vi "Reset.vi"(8 "error in (no error)":errorcluster, 10 "Set Defaults? (F)":bool, 11 "VISA resource name":refnum<visa-resource-name>) -> (0 "error out":errorcluster, 3 "VISA resource name out":refnum<visa-resource-name>)   [LabVIEW 2011, in "MGC647C.lvlib"]
doc: "Resets the instrument and then sends a set of default setup commands to the instrument."
uses:
  <instrlib>/MGC647C/MGC647C.lvlib
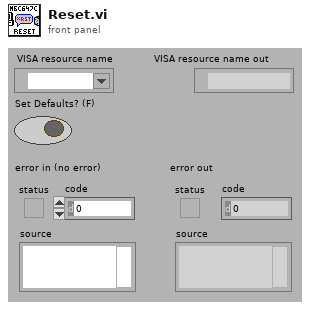
[diagram p1: front panel]
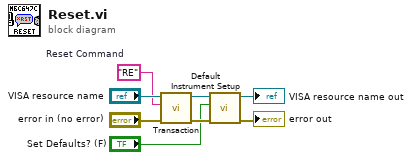
[diagram p0: block diagram]
diagram:
  w2 = "RE"  # Reset Command
  n1 = call <instrlib>:"Transaction.vi"("Error In"="error in (no error)", "Command"=w2, "VISA resource name"="VISA resource name") -> ("Error Out"=w5:errorcluster, "dup VISA resource name"=w6:refnum<visa-resource-name>)  [unwired: 6 in, 1 out]
  n2 = call <instrlib>:"Default Instrument Setup.vi"("error in (no error)"=w5, "Set Defaults? (F)"="Set Defaults? (F)", "VISA resource name"=w6) -> ("error out"=→"error out":errorcluster, "VISA resource name out"=→"VISA resource name out":refnum<visa-resource-name>)  [unwired: 7 in]
